vi "Error Code to String.vi"(10 "Code":dbl caption="代码") -> (2 "Info String":string caption="信息")   [LabVIEW 2023, in "Longer Pump dLSP501 Series.lvlib"]
uses:
  <instrlib>/Longer Pump dLSP501 Modbus RTU Series/Longer Pump dLSP501 Series.lvlib
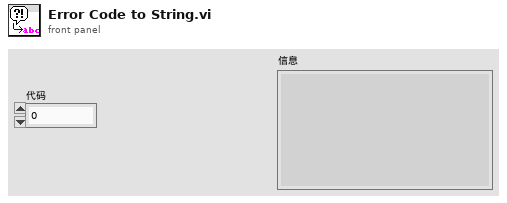
[diagram p1: front panel]
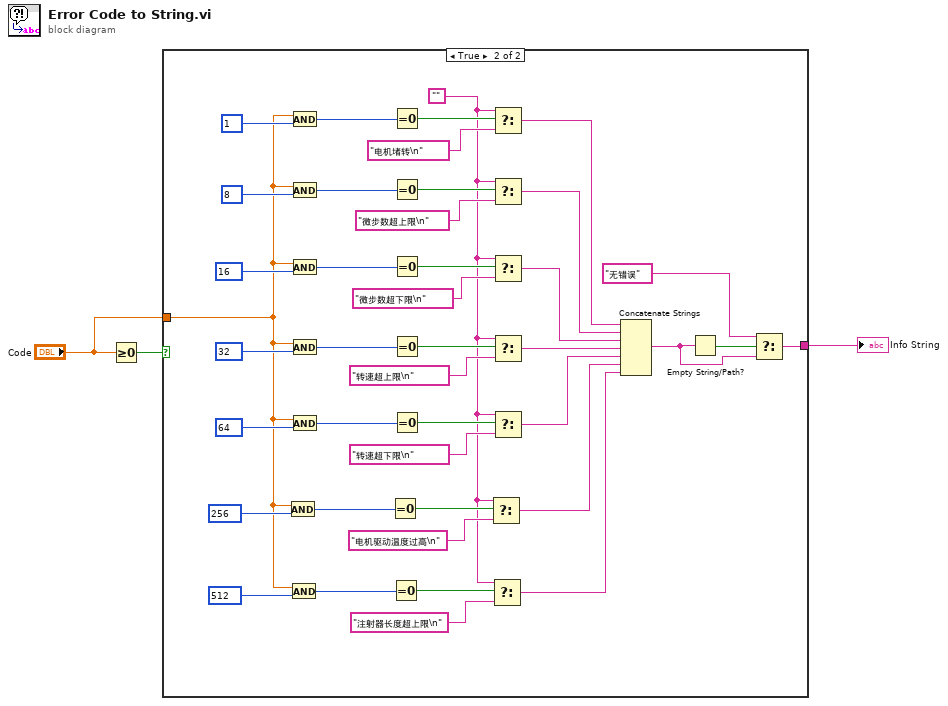
[diagram p0: block diagram]
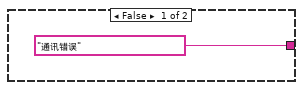
[diagram p2: hidden frame]
diagram:
  n1 = Greater Or Equal To 0?(x="Code") -> (x >= 0?=w3:bool)
  n2 = case shown="True" w3 {
    tunnel: ["通讯错误" ("Status 2") w14] -> w2
    tunnel: "Code" -> [_ w5]
    frame False {
    }
    frame True {
      w6 = ""
      n3 = And(x=w5, y=u32 256) -> (x .and. y?=w19:i32)
      n4 = And(x=w5, y=u32 512) -> (x .and. y?=w10:i32)
      n5 = And(x=w5, y=u32 1) -> (x .and. y?=w44:i32)
      n6 = And(x=w5, y=u32 8) -> (x .and. y?=w39:i32)
      n7 = And(x=w5, y=u32 16) -> (x .and. y?=w34:i32)
      n8 = And(x=w5, y=u32 32) -> (x .and. y?=w30:i32)
      n9 = And(x=w5, y=u32 64) -> (x .and. y?=w26:i32)
      n10 = Equal To 0?(x=w19) -> (x = 0?=w18:bool)
      n11 = Equal To 0?(x=w10) -> (x = 0?=w9:bool)
      n12 = Equal To 0?(x=w44) -> (x = 0?=w43:bool)
      n13 = Equal To 0?(x=w39) -> (x = 0?=w38:bool)
      n14 = Equal To 0?(x=w34) -> (x = 0?=w33:bool)
      n15 = Equal To 0?(x=w30) -> (x = 0?=w29:bool)
      n16 = Equal To 0?(x=w26) -> (x = 0?=w25:bool)
      n17 = Select(t=w6, s=w18, f="电机驱动温度过高\n" ("Status 2")) -> (s? t:f=w16:string)
      n18 = Select(t=w6, s=w9, f="注射器长度超上限\n" ("Status 2")) -> (s? t:f=w7:string)
      n19 = Select(t=w6, s=w43, f="电机堵转\n" ("Status 2")) -> (s? t:f=w41:string)
      n20 = Select(t=w6, s=w38, f="微步数超上限\n" ("Status 2")) -> (s? t:f=w36:string)
      n21 = Select(t=w6, s=w33, f="微步数超下限\n" ("Status 2")) -> (s? t:f=w23:string)
      n22 = Select(t=w6, s=w29, f="转速超上限\n" ("Status 2")) -> (s? t:f=w21:string)
      n23 = Select(t=w6, s=w25, f="转速超下限\n" ("Status 2")) -> (s? t:f=w22:string)
      n24 = Concatenate Strings(w41, w36, w23, w21, w22, w16, w7) -> (w15:string)
      n25 = Empty String/Path?(string/path=w15) -> (empty?=w13:bool)
      n26 = Select(t="无错误", s=w13, f=w15) -> (s? t:f=w14:string)
    }
  }
  "Info String" <- w2
